vi "DetConnect-com-exec.vi"(8 "error in (no error)":errorcluster, 9 "data":variant, 10 "ControlQueue":refnum<queue>, 11 "Detector in":refnum<class "Detector.lvclass">) -> (0 "error out":errorcluster, 2 "BG_level":i32, 3 "Detector out":refnum<class "Detector.lvclass">)   [LabVIEW 2020, in "Detector.lvclass"]
uses:
  Detector.lvclass
  dependecies/ControlsVIs/Clusters-def/SERVER-Commands.ctl
  dependecies/ControlsVIs/Clusters-def/Det-Reply-to-Connect-client.ctl
  dependecies/ControlsVIs/Clusters-def/Det-Reply-to-Connect.ctl
  Detector.lvclass/Detector.ctl
  Control/Control-Server/Control-Server.lvclass
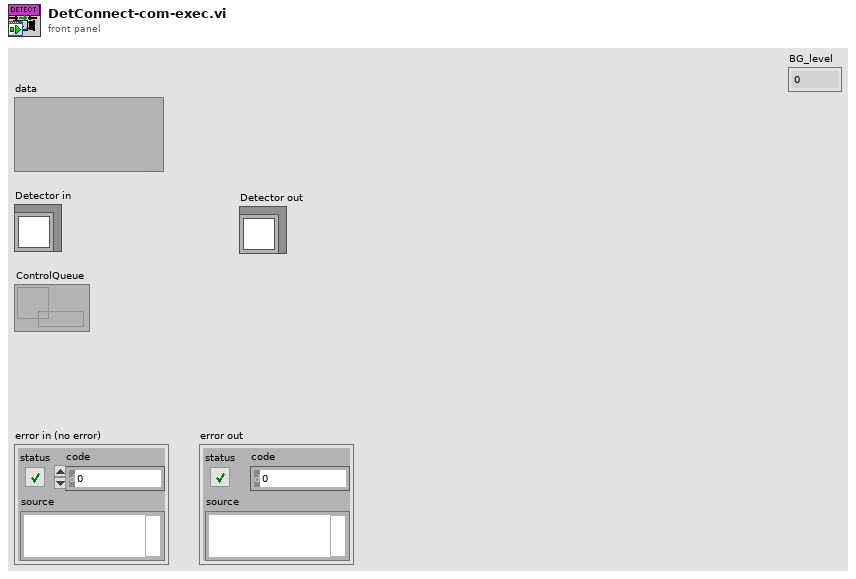
[diagram p1: front panel]
types:
  T1 = typedef "Control-Server.lvclass/SERVER-Commands.ctl" = string
  T2 = typedef "Detector.lvclass/Det-Reply-to-Connect.ctl" = cluster{"On/Off":bool, "error":errorcluster, "Detector":refnum<class "Detector.lvclass">}
  T3 = typedef "Detector.lvclass/Det-Reply-to-Connect-client.ctl" = cluster{"on/off":bool, "calibration":dbl[], "error":errorcluster}
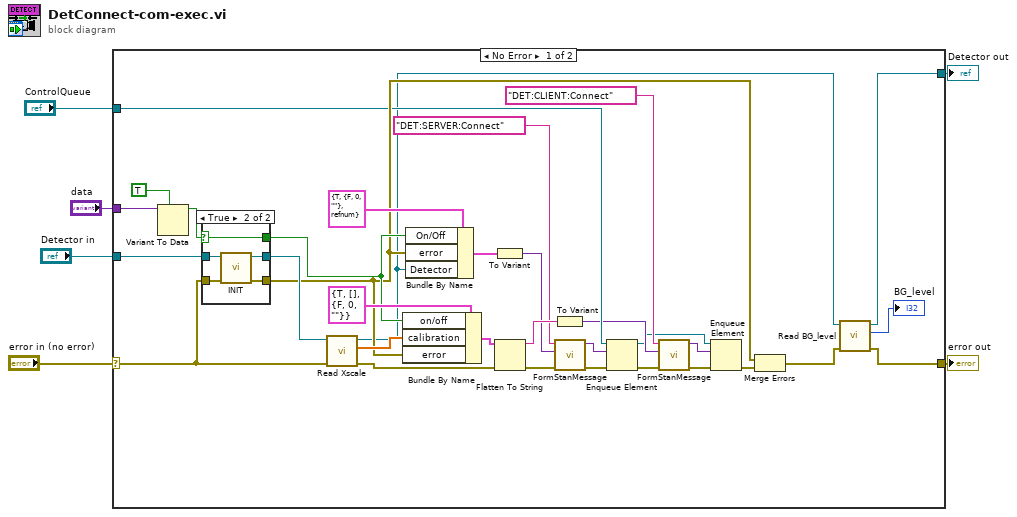
[diagram p0: block diagram]
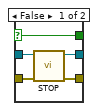
[diagram p2: hidden frame]
diagram:
  n1 = case shown="No Error" "error in (no error)" {
    selector: "error in (no error)" -> [w26 w51]
    tunnel: "data" -> [w39 _]
    tunnel: [w9 w50] -> w5
    tunnel: "Detector in" -> [w38 w50]
    tunnel: "ControlQueue" -> [w17 _]
    tunnel: [w11 w51] -> w2
    frame No Error {
      n2 = Variant To Data(type=TRUE, Variant=w39) -> (data=w28:bool)  [unwired: 1 in, 1 out]
      n3 = case shown="True" w28 {
        selector: w28 -> [w41 w46]
        tunnel: [w43 w49] -> w30
        tunnel: w38 -> [w44 w48]
        tunnel: [w42 w47] -> w27
        tunnel: [w41 w46] -> w31
        tunnel: w26 -> [w40 w45]
        frame False {
          n4 = call-dynamic "STOP.vi"("error in (no error)"=w40, "Stop in"=w44) -> ("error out"=w42:errorcluster, "Stop out"=w43:refnum<class "Detector.lvclass">)  [unwired: 8 in]
        }
        frame True {
          n5 = call-dynamic "INIT.vi"("error in (no error)"=w45, "Detector in"=w48) -> ("error out"=w47:errorcluster, "Detector out"=w49:refnum<class "Detector.lvclass">)  [unwired: 8 in]
        }
      }
      n6 = call "Read Xscale.vi"("error in (no error)"=w26, "Detector en entrée"=w30) -> ("error out"=w25:errorcluster, "Xscale"=w36:dbl[], "Detector en sortie"=w10:refnum<class "Detector.lvclass">)  [unwired: 7 in]
      n7 = Bundle By Name(cluster=T3 {"on/off"=TRUE, "calibration"=[], "error"={"status"=FALSE, "code"=0, "source"=""}}, "on/off"=w31, "calibration"=w36, "error"=w27) -> (w35:T3)
      n8 = Bundle By Name(cluster=T2 {"On/Off"=TRUE, "error"={"status"=FALSE, "code"=0, "source"=""}, "Detector"=refnum} ("Cluster"), "On/Off"=w31, "error"=w27, "Detector"=w10) -> (w32:T2)
      n9 = To Variant(anything=w32) -> (Variant=w15:variant)
      n10 = Flatten To String(anything=w35, error in (no error)=w25) -> (data string=w34:string, error out=w24:errorcluster)  [unwired: 2 in, 1 out]
      n11 = To Variant(anything=w34) -> (Variant=w13:variant)
      n12 = call "FormStanMessage.vi"("error in"=w24, "data"=w15, "Command"=T1 "DET:SERVER:Connect" ("Commands")) -> ("error out"=w23:errorcluster, "message"=w22:variant)  [unwired: 7 in]
      n13 = Enqueue Element(queue=w17, element=w22, error in (no error)=w23) -> (queue out=w7:refnum<queue>, error out=w20:errorcluster)  [unwired: 1 in, 1 out]
      n14 = call "FormStanMessage.vi"("error in"=w20, "data"=w13, "Command"=T1 "DET:CLIENT:Connect" ("Commands")) -> ("error out"=w19:errorcluster, "message"=w14:variant)  [unwired: 7 in]
      n15 = Enqueue Element(queue=w7, element=w14, error in (no error)=w19) -> (error out=w18:errorcluster)  [unwired: 1 in, 2 out]
      n16 = Merge Errors(w27, w18) -> (w12:errorcluster)
      n17 = call-dynamic "Read BG_level.vi"("error in (no error)"=w12, "Detector in"=w10) -> ("error out"=w11:errorcluster, "BG_level"=→"BG_level":i32, "Detector out"=w9:refnum<class "Detector.lvclass">)  [unwired: 7 in]
    }
    frame Error {
    }
  }
  "error out" <- w2
  "Detector out" <- w5
